vi "Write.vi"(0 "reference in":refnum<class "Torque.lvclass">, 5 "error in (no error)":errorcluster) -> (14 "reference out":refnum<class "Torque.lvclass">, 19 "error out":errorcluster)   [LabVIEW 2013, in "Torque.lvclass"]
uses:
  Torque.lvclass
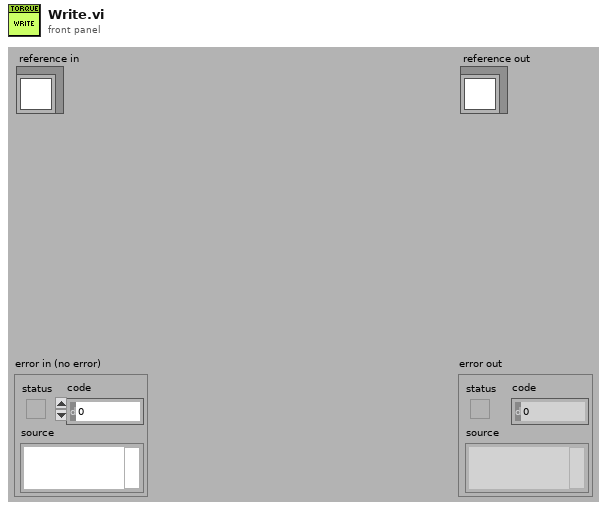
[diagram p1: front panel]
types:
  T1 = typedef "Torque.lvclass/ObjectAttributes.ctl" = cluster{"MyAttribute":dbl}
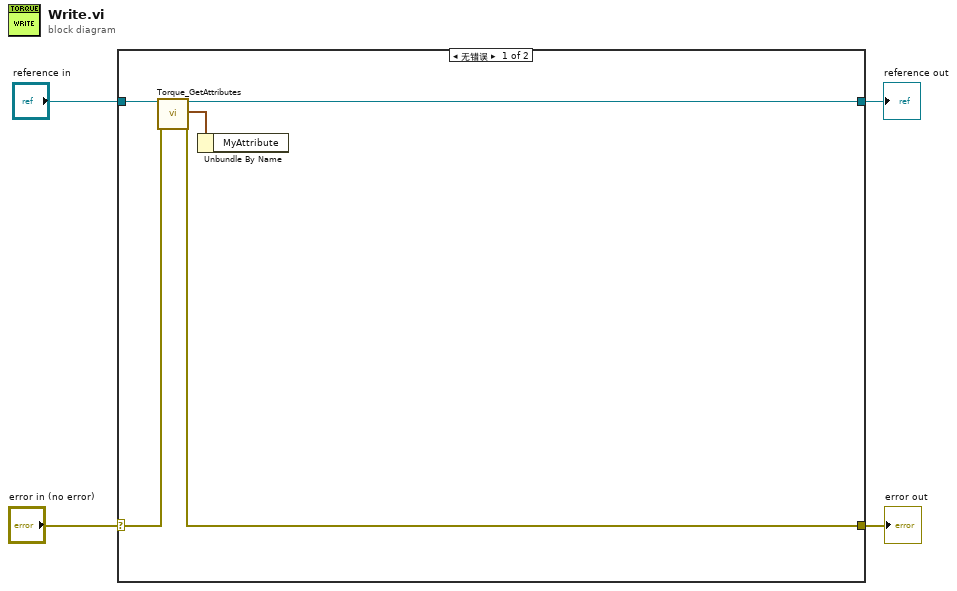
[diagram p0: block diagram]
diagram:
  n1 = case shown="无错误" "error in (no error)" {
    selector: "error in (no error)" -> [w9 w11]
    tunnel: [w8 w11] -> w3
    tunnel: [w7 w10] -> w1
    tunnel: "reference in" -> [w5 w10]
    frame No Error {
      n2 = call "Torque_GetAttributes.vi"("reference in"=w5, "error in (no error)"=w9) -> ("reference out"=w7:refnum<class "Torque.lvclass">, "attributes"=w6:T1, "error out"=w8:errorcluster)  [unwired: 14 in, 1 out]
      n3 = Unbundle By Name(w6) -> ()  [unwired: 1 out]
    }
    frame Error {
    }
  }
  "error out" <- w3
  "reference out" <- w1
